vi "render hold note.vi"(4 "head index":i32, 6 "progress":dbl, 7 "y-center":dbl, 9 "head position":dbl, 10 "rail":cluster{"note type":string, "position":dbl}[](array[cluster]), 11 "new picture in":picture) -> (3 "new picture out":picture)   [LabVIEW 2023]
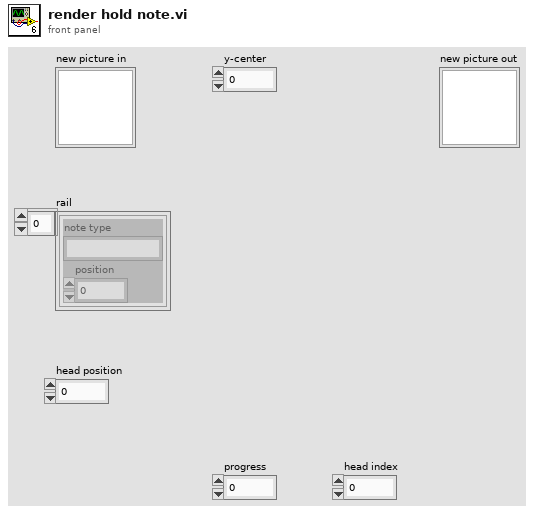
[diagram p1: front panel]
types:
  T1 = cluster{"Width":u16, "Style":enum32{"Solid", "Dash", "Dot", "DashDot", "DashDotDot"}}
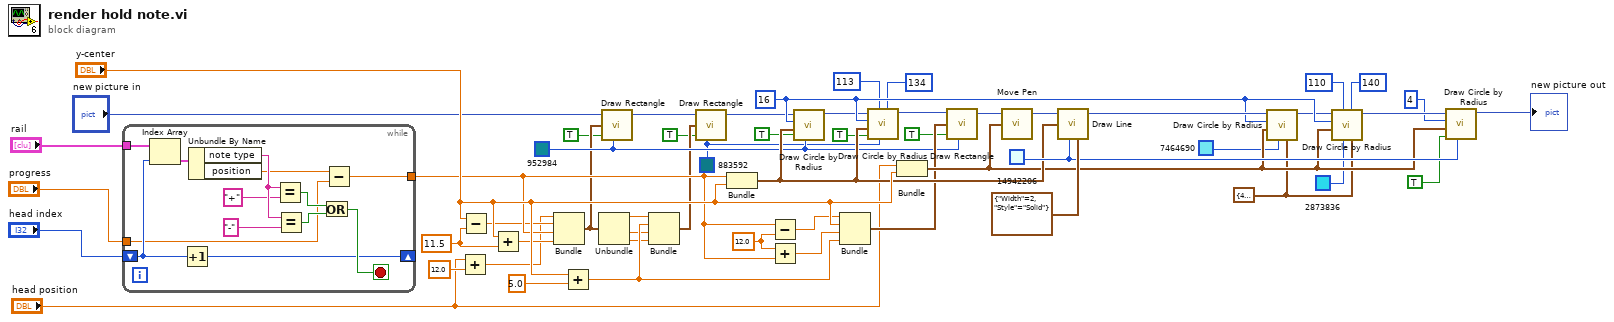
[diagram p0: block diagram]
diagram:
  w41 = 12.0 ("y")
  w33 = u32 883592 ("color(black)")
  w52 = u32 14942206 ("color(black)")
  w40 = u32 952984 ("color(black)")
  w18 = 11.5 ("y")
  w6 = T1 {"Width"=4, "Style"=enum."Solid"} ("pen")
  w37 = i16 16 ("radius")
  n1 = while {
    tunnel: "rail" -> [w67]
    shift-right: [w58] -> _
    shift-left: "head index" -> [w59]
    tunnel: "progress" -> [w57]
    tunnel: [w55] -> w42
    stop <- w60 stop-if-true
    n2 = Index Array(array=w67, index=w59) -> (element=w66:cluster{"note type":string, "position":dbl})
    n3 = Increment(x=w59) -> (x+1=w58:i32)
    n4 = Unbundle By Name(w66) -> ("note type"=w63:string, "position"=w56:dbl)
    n5 = Equal?(x=w63, y="+") -> (x = y?=w65:bool)
    n6 = Equal?(x=w63, y="-") -> (x = y?=w64:bool)
    n7 = Or(x=w65, y=w64) -> (x .or. y?=w60:bool)
    n8 = Subtract(x=w56, y=w57) -> (x-y=w55:dbl)
  }
  n9 = Add(x="head position", y=12.0) -> (x+y=w16:dbl)
  n10 = Subtract(x="y-center", y=w18) -> (x-y=w17:dbl)
  n11 = Add(x="y-center", y=w18) -> (x+y=w19:dbl)
  n12 = Bundle(w16, w17, w42, w19) -> (w26:cluster{dbl, dbl, dbl, dbl})  [unwired: 1 in]
  n13 = Add(x="y-center", y=5.0) -> (x+y=w45:dbl)
  n14 = Unbundle(w26) -> (w27:dbl, w28:dbl, w29:dbl)  [unwired: 1 out]
  n15 = call <vilib>:"Draw Rectangle.vi"("picture"="new picture in", "rect"=w26, "fill?(F)"=TRUE, "color(black)"=w40) -> ("new picture"=w23:picture)  [unwired: 5 in]
  n16 = Bundle(w27, w45, w28, w29) -> (w31:cluster{dbl, dbl, dbl, dbl})  [unwired: 1 in]
  n17 = call <vilib>:"Draw Rectangle.vi"("picture"=w23, "rect"=w31, "fill?(F)"=TRUE, "color(black)"=w33) -> ("new picture"=w24:picture)  [unwired: 5 in]
  n18 = Bundle(w42, "y-center"="y-center") -> (w50:cluster{dbl, "y-center":dbl})  [unwired: 1 in]
  n19 = Subtract(x=w42, y=w41) -> (x-y=w43:dbl)
  n20 = Add(x=w41, y=w42) -> (x+y=w44:dbl)
  n21 = call <vilib>:"Draw Circle by Radius.vi"("color(black)"=w40, "fill?(F)"=TRUE, "pixel center"=w50, "radius"=w37, "picture"=w24) -> ("new picture"=w32:picture)  [unwired: 6 in]
  n22 = Bundle(w43, "y-center"="y-center", w44, w45) -> (w46:cluster{dbl, "y-center":dbl, dbl, dbl})  [unwired: 1 in]
  n23 = call <vilib>:"Draw Circle by Radius.vi"("arc size(360)"=i16 134 ("radius"), "color(black)"=w33, "start angle(0)"=i16 113 ("radius"), "fill?(F)"=TRUE, "pixel center"=w50, "radius"=w37, "picture"=w32) -> ("new picture"=w38:picture)  [unwired: 4 in]
  n24 = Bundle("head position"="head position", "y-center"="y-center") -> (w48:cluster{"head position":dbl, "y-center":dbl})  [unwired: 1 in]
  n25 = call <vilib>:"Draw Rectangle.vi"("picture"=w38, "rect"=w46, "fill?(F)"=TRUE, "color(black)"=w40) -> ("new picture"=w47:picture)  [unwired: 5 in]
  n26 = call <vilib>:"Move Pen.vi"("new position"=w48, "picture"=w47) -> ("new picture"=w49:picture)  [unwired: 3 in]
  n27 = call <vilib>:"Draw Line.vi"("picture"=w49, "end point"=w50, "color(black)"=w52, "pen"=T1 {"Width"=2, "Style"=enum."Solid"}) -> ("new picture"=w51:picture)  [unwired: 5 in]
  n28 = call <vilib>:"Draw Circle by Radius.vi"("pen"=w6, "color(black)"=u32 7464690, "pixel center"=w48, "radius"=w37, "picture"=w51) -> ("new picture"=w4:picture)  [unwired: 6 in]
  n29 = call <vilib>:"Draw Circle by Radius.vi"("pen"=w6, "arc size(360)"=i16 140 ("radius"), "color(black)"=u32 2873836, "start angle(0)"=i16 110 ("radius"), "pixel center"=w48, "radius"=w37, "picture"=w4) -> ("new picture"=w5:picture)  [unwired: 4 in]
  n30 = call <vilib>:"Draw Circle by Radius.vi"("color(black)"=w52, "fill?(F)"=TRUE, "pixel center"=w48, "radius"=i16 4, "picture"=w5) -> ("new picture"=→"new picture out":picture)  [unwired: 6 in]
